vi "Close.vi"(8 "error in":errorcluster, 11 "DB-MySQL in":refnum<class "DB-MySQL.lvclass">=refnum) -> (0 "error out":errorcluster, 3 "DB-MySQL out":refnum<class "DB-MySQL.lvclass">)   [LabVIEW 2014, in "hse-db.lvlib" / "DB-MySQL.lvclass"]
uses:
  DB-MySQL.lvclass
  DB-MySQL.lvclass/DB-MySQL.ctl
  DB-Engines/MySQLTcp/MySQL (TCP).lvlib
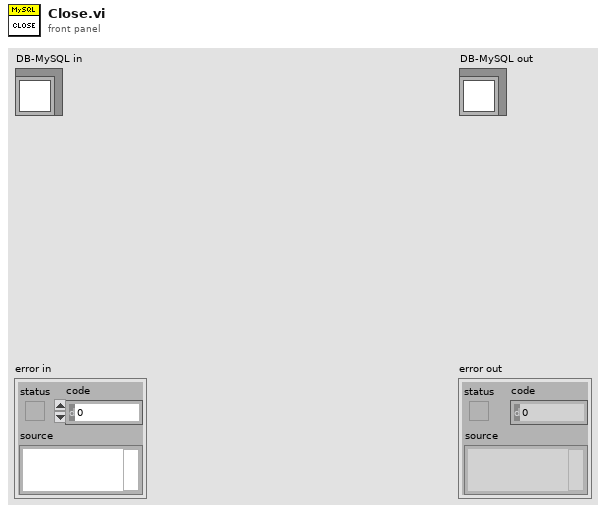
[diagram p1: front panel]
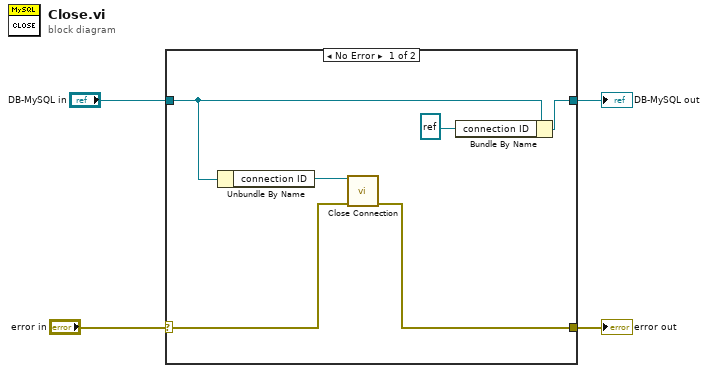
[diagram p0: block diagram]
diagram:
  n1 = case shown="No Error" "error in" {
    selector: "error in" -> [w7 w11]
    tunnel: [w6 w11] -> w3
    tunnel: [w9 w12] -> w1
    tunnel: "DB-MySQL in" -> [w10 w12]
    frame No Error {
      n2 = Unbundle By Name(w10) -> ("connection ID"=w5:refnum<k5>)
      n3 = call "Close Connection.vi"("connection ID"=w5, "error in (no error)"=w7) -> ("error out"=w6:errorcluster)  [unwired: 13 in]
      n4 = Bundle By Name(cluster=w10, "connection ID"=refnum<k5> refnum) -> (w9:refnum<class "DB-MySQL.lvclass">)
    }
    frame Error {
    }
  }
  "error out" <- w3
  "DB-MySQL out" <- w1
